vi "Atividade 4.vi"() -> ()   [LabVIEW 2015]
uses:
  <vilib>/Analysis/baseanly.llb/Mean (DBL).vi
  <vilib>/express/express shared/transition.llb/Dynamic To Waveform Array.vi
  <vilib>/express/express arith-compare/Formula/Block/exnFormulaBlock how many pts in the wave.vi
  <vilib>/express/express shared/ex_Modify Signal Name.vi
  <vilib>/express/express shared/transition.llb/Waveform Array To Dynamic.vi
  <vilib>/express/express arith-compare/Formula/XNode/ExpressFormulaBlockNode.xnode
  <vilib>/Analysis/NI_AALBase.lvlib
panel:
  out "Temperatura":dbl
  out "Tensao eletrica":dbl
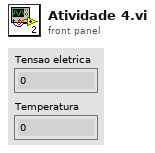
[diagram p1: front panel]
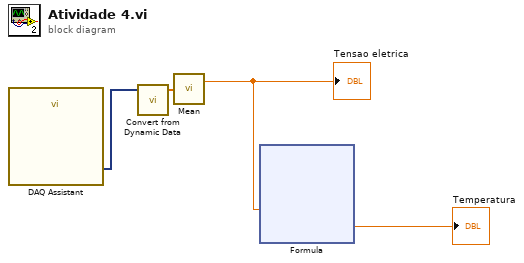
[diagram p0: block diagram]
diagram:
  n1 = call "DAQ Assistant"() -> ("data"=w2:dynamicdata)  [unwired: 17 in, 2 out]
  n2 = call "Convert from Dynamic Data"("Dynamic Data Type"=w2) -> ("Array"=w4:dbl[])  [unwired: 3 in]
  n3 = call-poly <vilib>:"Mean.vi"("X"=w4) -> ("mean"=w1:dbl)  [unwired: 1 out]
  "Tensao eletrica" <- w1
  n4 = xnode "Formula"("V"=w1) -> ("Result"=→"Temperatura":dbl)  [unwired: 1 in, 1 out]
